vi "Initialize Analyzer from Experiment Cluster.vi"(8 "error in (no error)":errorcluster, 11 "Reaction Rover Data":T1={"Visible Hardware VI"="", "Current Message"={"Source"="", "Destination"="", "Time Stamp"=timestamp(0 s since 1904-01-01), "Command"="", "Data"=variant(string "")}, "Message History"=[], "Hardware"={"Process Cache"=refnum, "Plugins"=[{"Plugin Name"="", "Controller Type"=enum."Invalid", "Control Panel Path"=path "", "Plugin Type"=enum."Optimizer", "Config Errors"=[]}, {"Plugin Name"="", "Controller Type"=enum."Invalid", "Control Panel Path"=path "", "Plugin Type"=enum."Optimizer", "Config Errors"=[]}, {"Plugin Name"="", "Controller Type"=enum."Invalid", "Control Panel Path"=path "", "Plugin Type"=enum."Optimizer", "Config Errors"=[]}, {"Plugin Name"="", "Controller Type"=enum."Invalid", "Control Panel Path"=path "", "Plugin Type"=enum."Optimizer", "Config Errors"=[]}]}, "Optimizers"={"Process Cache"=refnum, "Plugins"=[{"Plugin Name"="", "Controller Type"=enum."Invalid", "Control Panel Path"=path "", "Plugin Type"=enum."Optimizer", "Config Errors"=[]}, {"Plugin Name"="", "Controller Type"=enum."Invalid", "Control Panel Path"=path "", "Plugin Type"=enum."Optimizer", "Config Errors"=[]}, {"Plugin Name"="", "Controller Type"=enum."Invalid", "Control Panel Path"=path "", "Plugin Type"=enum."Optimizer", "Config Errors"=[]}], "First parameteres?"=FALSE, "New Parameters"={"Time Stamp"=timestamp(0 s since 1904-01-01), "Names"=[], "Values"=[]}}, "Parameter to Hardware Map"=refnum, "Analyzers"={"Process Cache"=refnum, "Plugins"=[{"Plugin Name"="", "Controller Type"=enum."Invalid", "Control Panel Path"=path "", "Plugin Type"=enum."Optimizer", "Config Errors"=[]}, {"Plugin Name"="", "Controller Type"=enum."Invalid", "Control Panel Path"=path "", "Plugin Type"=enum."Optimizer", "Config Errors"=[]}, {"Plugin Name"="", "Controller Type"=enum."Invalid", "Control Panel Path"=path "", "Plugin Type"=enum."Optimizer", "Config Errors"=[]}, {"Plugin Name"="", "Controller Type"=enum."Invalid", "Control Panel Path"=path "", "Plugin Type"=enum."Optimizer", "Config Errors"=[]}]}, "Log Directory"=path "", "Auto Pass Parameters"=FALSE, "Experiment"={"Name"="", "File Path"=path "", "File Extension"="", "File Cluster"={"Hardware List"=[], "Optimizer List"=[], "Analyzer List"=[], "Parameter to Hardware Map"=[]}}, "Main VI Queue"=refnum, "Process Queue References"=[], "Message Queue"=refnum, "User Preferences File"=refnum}) -> (0 "error out":errorcluster, 2 "Load Success":bool[](array[boolean]), 3 "Reaction Rover Data out":T1={"Visible Hardware VI"="", "Current Message"={"Source"="", "Destination"="", "Time Stamp"=timestamp(0 s since 1904-01-01), "Command"="", "Data"=variant(string "")}, "Message History"=[], "Hardware"={"Process Cache"=refnum, "Plugins"=[{"Plugin Name"="", "Controller Type"=enum."Invalid", "Control Panel Path"=path "", "Plugin Type"=enum."Optimizer", "Config Errors"=[]}, {"Plugin Name"="", "Controller Type"=enum."Invalid", "Control Panel Path"=path "", "Plugin Type"=enum."Optimizer", "Config Errors"=[]}, {"Plugin Name"="", "Controller Type"=enum."Invalid", "Control Panel Path"=path "", "Plugin Type"=enum."Optimizer", "Config Errors"=[]}, {"Plugin Name"="", "Controller Type"=enum."Invalid", "Control Panel Path"=path "", "Plugin Type"=enum."Optimizer", "Config Errors"=[]}]}, "Optimizers"={"Process Cache"=refnum, "Plugins"=[{"Plugin Name"="", "Controller Type"=enum."Invalid", "Control Panel Path"=path "", "Plugin Type"=enum."Optimizer", "Config Errors"=[]}, {"Plugin Name"="", "Controller Type"=enum."Invalid", "Control Panel Path"=path "", "Plugin Type"=enum."Optimizer", "Config Errors"=[]}, {"Plugin Name"="", "Controller Type"=enum."Invalid", "Control Panel Path"=path "", "Plugin Type"=enum."Optimizer", "Config Errors"=[]}], "First parameteres?"=FALSE, "New Parameters"={"Time Stamp"=timestamp(0 s since 1904-01-01), "Names"=[], "Values"=[]}}, "Parameter to Hardware Map"=refnum, "Analyzers"={"Process Cache"=refnum, "Plugins"=[{"Plugin Name"="", "Controller Type"=enum."Invalid", "Control Panel Path"=path "", "Plugin Type"=enum."Optimizer", "Config Errors"=[]}, {"Plugin Name"="", "Controller Type"=enum."Invalid", "Control Panel Path"=path "", "Plugin Type"=enum."Optimizer", "Config Errors"=[]}, {"Plugin Name"="", "Controller Type"=enum."Invalid", "Control Panel Path"=path "", "Plugin Type"=enum."Optimizer", "Config Errors"=[]}, {"Plugin Name"="", "Controller Type"=enum."Invalid", "Control Panel Path"=path "", "Plugin Type"=enum."Optimizer", "Config Errors"=[]}]}, "Log Directory"=path "", "Auto Pass Parameters"=FALSE, "Experiment"={"Name"="", "File Path"=path "", "File Extension"="", "File Cluster"={"Hardware List"=[], "Optimizer List"=[], "Analyzer List"=[], "Parameter to Hardware Map"=[]}}, "Main VI Queue"=refnum, "Process Queue References"=[], "Message Queue"=refnum, "User Preferences File"=refnum})   [LabVIEW 2020, in "RxnRover.lvlib"]
uses:
  RxnRover.lvlib
  Type Definitions/Data.ctl
  Plugin Servers/Parameter to Hardware Map/Parameter to Hardware Map.lvclass
  User Preferences/User Preferences File.lvclass
  <userlib>/RxnRover/DynamicReentrant/src/Type Defs/Message.ctl
  Plugin Details.ctl
  Plugin Servers/Controller/Controller Type.ctl
  Plugin Types.ctl
  Config Error.ctl
  Type Definitions/New Parameters.ctl
  Experiment/Experiment File/Experiment File Cluster.ctl
  Plugin Servers/Controller/Minimal Controller Cluster.ctl
  Plugin Servers/Parameter to Hardware Map/Minimal Map.ctl
  Plugin Servers/Parameter to Hardware Map/Minimal Pair Cluster.ctl
  Plugin Servers/Controller/Generic Plugin.lvclass/Generic Plugin.ctl
  <userlib>/RxnRover/DynamicReentrant/Dynamic Reentrant.lvlib
  Plugin Servers/Controller/Generic Plugin.lvclass
  Plugin Servers/Controller Array/Controller Array.lvclass
  Experiment/Experiment File/Experiment File.lvlib
  Plugin Manager.lvlib
panel:
  # "Note: Rxn Rover data control and indicator are hidden!"
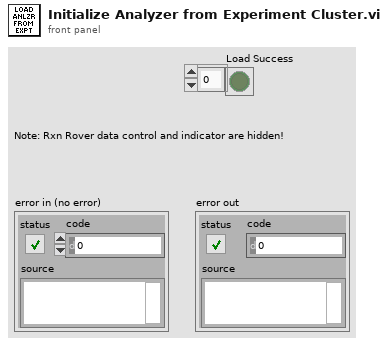
[diagram p1: front panel]
types:
  T1 = typedef "RxnRover.lvlib/Data.ctl" = cluster{"Visible Hardware VI":string, "Current Message":T2, "Message History":string[][], "Hardware":cluster{"Process Cache":refnum<class "Controller Array.lvclass">, "Plugins":T3[]}, "Optimizers":cluster{"Process Cache":refnum<class "Controller Array.lvclass">, "Plugins":T3[], "First parameteres?":bool, "New Parameters":T7}, "Parameter to Hardware Map":refnum<class "Parameter to Hardware Map.lvclass">, "Analyzers":cluster{"Process Cache":refnum<class "Controller Array.lvclass">, "Plugins":T3[]}, "Log Directory":path, "Auto Pass Parameters":bool, "Experiment":cluster{"Name":string, "File Path":path, "File Extension":string, "File Cluster":T8}, "Main VI Queue":refnum<queue>, "Process Queue References":refnum<queue>[], "Message Queue":refnum<queue>, "User Preferences File":refnum<class "User Preferences File.lvclass">}
  T2 = typedef "Dynamic Reentrant.lvlib/Message.ctl" = cluster{"Source":string, "Destination":string, "Time Stamp":timestamp, "Command":string, "Data":variant}
  T3 = typedef "RxnRover.lvlib/Plugin Manager.lvlib/Plugin Details.ctl" = cluster{"Plugin Name":string, "Controller Type":T4, "Control Panel Path":path, "Plugin Type":T5, "Config Errors":T6[]}
  T4 = typedef "RxnRover.lvlib/Generic Plugin.lvclass/Controller Type.ctl" = enum16{"Invalid", "Temperature Controller", "Pump Controller", "Syringe Pump", "Generic Optimizer", "LC Parser", "Passive Hardware"}
  T5 = typedef "RxnRover.lvlib/Plugin Manager.lvlib/Plugin Types.ctl" = enum16{"Invalid", "Optimizer", "Analyzer", "Hardware"}
  T6 = typedef "RxnRover.lvlib/Plugin Manager.lvlib/Config Error.ctl" = cluster{"Error?":bool, "Message":string}
  T7 = typedef "RxnRover.lvlib/New Parameters.ctl" = cluster{"Time Stamp":timestamp, "Names":string[], "Values":variant[]}
  T8 = typedef "RxnRover.lvlib/Experiment File.lvlib/Experiment File Cluster.ctl" = cluster{"Hardware List":T9[], "Optimizer List":T9[], "Analyzer List":T9[], "Parameter to Hardware Map":T10}
  T9 = typedef "RxnRover.lvlib/Generic Plugin.lvclass/Minimal Controller Cluster.ctl" = cluster{"Name":string, "Controller Type":string, "Control Panel Path":string, "Resource":string}
  T10 = typedef "RxnRover.lvlib/Parameter to Hardware Map.lvclass/Minimal Map.ctl" = T11[]
  T11 = typedef "RxnRover.lvlib/Parameter to Hardware Map.lvclass/Minimal Pair Cluster.ctl" = cluster{"key":string, "values":T9[]}
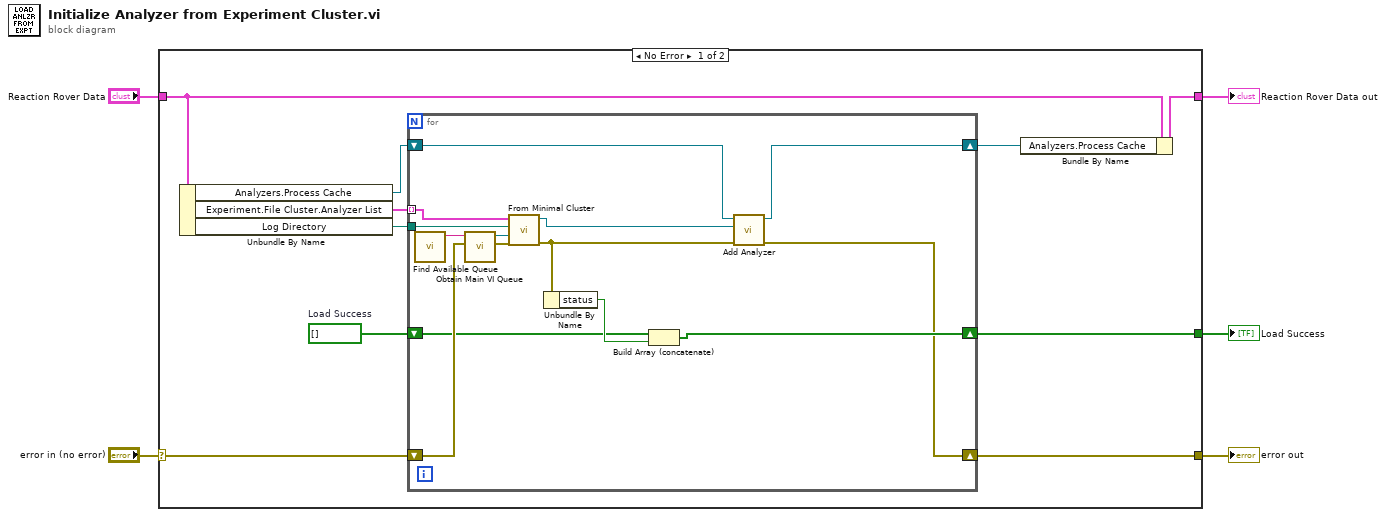
[diagram p0: block diagram]
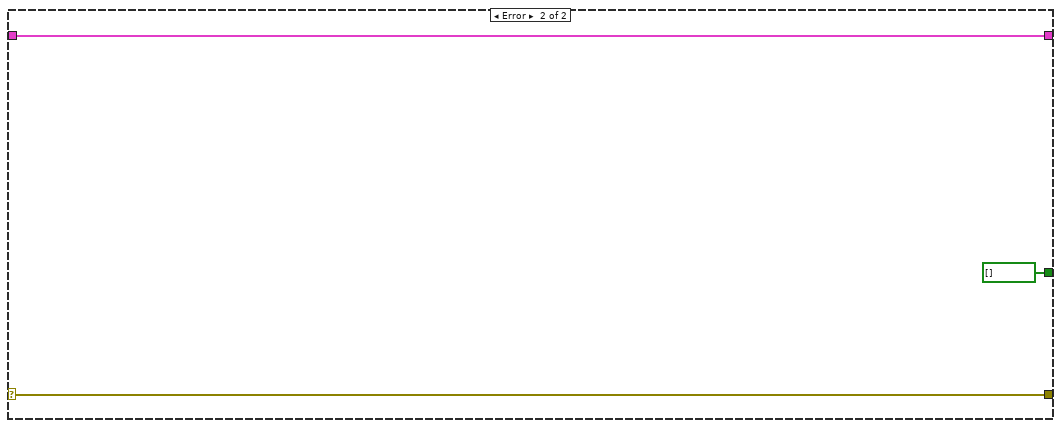
[diagram p2: hidden frame]
diagram:
  n1 = case shown="No Error" "error in (no error)" {
    selector: "error in (no error)" -> [w14 w32]
    tunnel: [w15 w32] -> w5
    tunnel: "Reaction Rover Data" -> [w13 w31]
    tunnel: [w11 w31] -> w2
    tunnel: [w6 bool[] [] ("Load Success")] -> w1
    frame No Error {
      w7 = bool[] []  # Load Success
      n2 = Unbundle By Name(w13) -> ("Analyzers.Process Cache"=w10:refnum<class "Controller Array.lvclass">, "Experiment.File Cluster.Analyzer List"=w9:T9[], "Log Directory"=w12:path)
      n3 = for {
        tunnel: w12 -> [w25]
        shift-right: [w19] -> w15
        shift-left: w14 -> [w26]
        shift-right: [w16] -> w8
        shift-left: w10 -> [w17]
        tunnel: w9 -> [w24] mode=indexing
        shift-right: [w20] -> w6
        shift-left: w7 -> [w21]
        n4 = call "Find Available Queue.vi"() -> ("String"=w29:string)  [unwired: 11 in]
        n5 = call <userlib>:"Obtain Main VI Queue.vi"("error in (no error)"=w26, "Name (Main VI)"=w29) -> ("error out"=w27:errorcluster, "Main VI Queue"=w28:refnum<queue>)  [unwired: 8 in]
        n6 = call "From Minimal Cluster.vi"("error in (no error)"=w27, "Receiving Queue"=w28, "Log Directory"=w25, "Minimal Controller Cluster"=w24) -> ("error out"=w23:errorcluster, "Plugin Server out"=w18:refnum<class "Generic Plugin.lvclass">)  [unwired: 6 in]
        n7 = Unbundle By Name(w23) -> ("status"=w22:bool)
        n8 = Build Array (concatenate)(w21, w22) -> (w20:bool[])
        n9 = call "Add Analyzer.vi"("error in (no error)"=w23, "new plugin"=w18, "Plugin Array in"=w17) -> ("error out"=w19:errorcluster, "Plugin Array out"=w16:refnum<class "Controller Array.lvclass">)  [unwired: 7 in]
      }
      n10 = Bundle By Name(cluster=w13, "Analyzers.Process Cache"=w8) -> (w11:T1)
    }
    frame Error {
    }
  }
  "error out" <- w5
  "Reaction Rover Data out" <- w2
  "Load Success" <- w1
